vi "FindTag.vi"(8 "error in (no error)":errorcluster, 10 "Tag":string, 11 "ToolStripItem":refnum<k24>) -> (0 "error out":errorcluster, 2 "Found":bool, 3 "ToolStripItem out":refnum<k24>)   [LabVIEW 2016, in "MGI_MenuStrip.lvclass"]
doc: "Authored by Derek E. Trepanier\nsupport@mooregoodideas.com\nwww.mooregoodideas.com\n\nCopyright (c) 2012, Moore Good Ideas, Inc.\n\nAll rights reserved.\n\nRedistribution and use in source and binary forms, with or without modification, are permitted provided that the following conditions are met:\n\n * Redistributions of source code must retain the above copyright notice, this list of conditions and the following disclaimer.\n * Redistributions in binary form must reproduce the above copyright notice, this list of conditions and the following disclaimer in the documentation and/or other materials provided with the distribution.\n * Neither the name of Moore Good Ideas, Inc. nor the names of its contributors may be used to endorse or promote products derived from this software without specific prior written permission.\n\nTHIS SOFTWARE IS PROVIDED BY THE COPYRIGHT HOLDERS AND CONTRIBUTORS \"AS IS\" AND ANY EXPRESS OR IMPLIED WARRANTIES, INCLUDING, BUT NOT LIMITED TO, THE IMPLIED WARRANTIES OF MERCHANTABILITY AND FITNESS FOR A PARTICULAR PURPOSE ARE DISCLAIMED. IN NO EVENT SHALL THE COPYRIGHT OWNER OR CONTRIBUTORS BE LIABLE FOR ANY DIRECT, INDIRECT, INCIDENTAL, SPECIAL, EXEMPLARY, OR CONSEQUENTIAL DAMAGES (INCLUDING, BUT NOT LIMITED TO, PROCUREMENT OF SUBSTITUTE GOODS OR SERVICES; LOSS OF USE, DATA, OR PROFITS; OR BUSINESS INTERRUPTION) HOWEVER CAUSED AND ON ANY THEORY OF LIABILITY, WHETHER IN CONTRACT, STRICT LIABILITY, OR TORT (INCLUDING NEGLIGENCE OR OTHERWISE) ARISING IN ANY WAY OUT OF THE USE OF THIS SOFTWARE, EVEN IF ADVISED OF THE POSSIBILITY OF SUCH DAMAGE."
uses:
  <userlib>/_MGI/Menu Building/MenuTypes/MenuStrip/MGI_MenuStrip.lvclass
  System.Windows.Forms
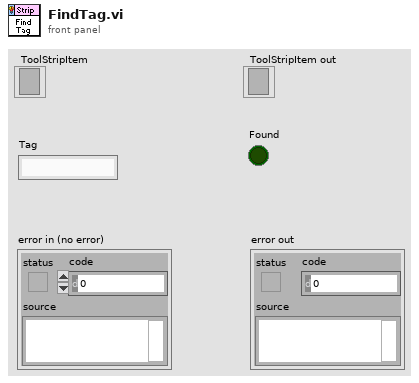
[diagram p1: front panel]
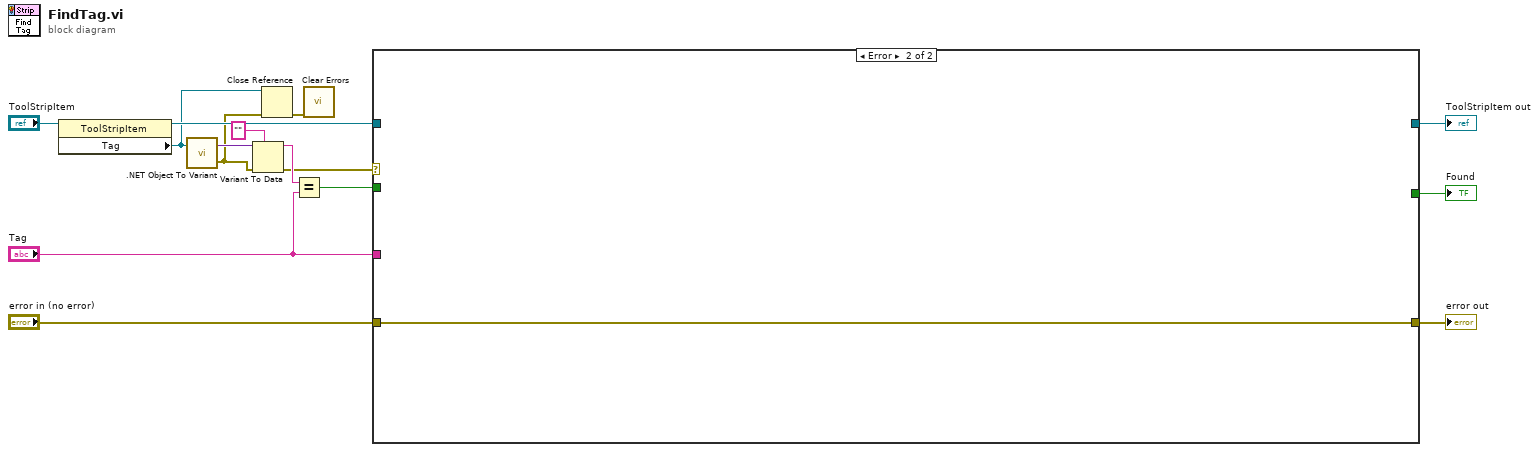
[diagram p0: block diagram]
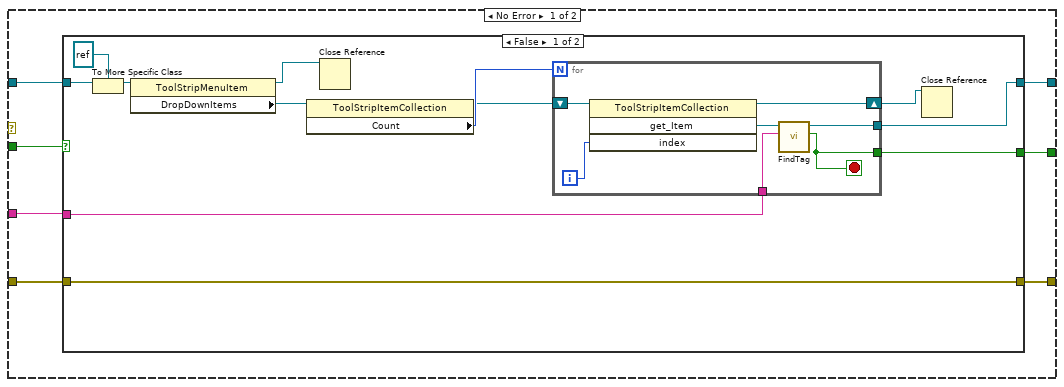
[diagram p2: hidden frame]
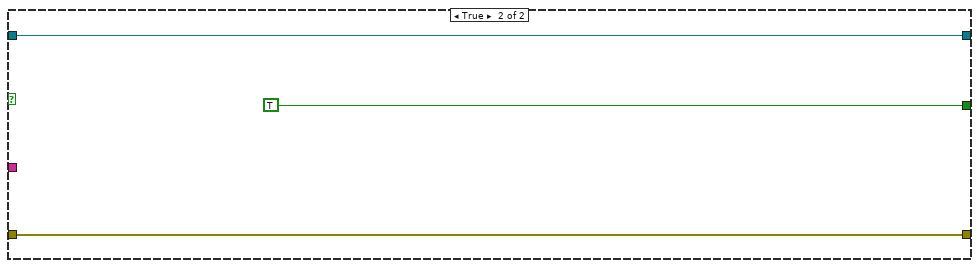
[diagram p3: hidden frame]
diagram:
  n1 = property class="ToolStripItem"(reference="ToolStripItem") -> (reference out=w9:refnum<k24>, "Tag"=w4:refnum<k24>)  [unwired: 1 in, 1 out]
  n2 = call <vilib>:".NET Object To Variant.vi"(".NET object"=w4) -> ("error out"=w3:errorcluster, "variant"=w14:variant)  [unwired: 1 in]
  n3 = Variant To Data(error in=w3, type="", Variant=w14) -> (data=w12:string, error out=w1:errorcluster)
  n4 = Close Reference(reference=w4, error in (no error)=w3) -> (error out=w2:errorcluster)
  n5 = Equal?(x=w12, y="Tag") -> (x = y?=w11:bool)
  n6 = call <vilib>:"Clear Errors.vi"("error in (no error)"=w2) -> ()  [unwired: 5 in, 2 out]
  n7 = case shown="Error" w1 {
    tunnel: w11 -> [w22 _]
    tunnel: [w21 _] -> w10
    tunnel: w9 -> [w20 _]
    tunnel: [w19 _] -> w8
    tunnel: [w18 w45] -> w7
    tunnel: "error in (no error)" -> [w17 w45]
    tunnel: "Tag" -> [w16 _]
    frame No Error {
      n8 = case shown="False" w22 {
        tunnel: [w27 w44] -> w21
        tunnel: w20 -> [w34 w44]
        tunnel: [w26 TRUE] -> w19
        tunnel: [w25 w42] -> w18
        tunnel: w17 -> [w25 w42]
        tunnel: w16 -> [w28 _]
        frame False {
          n9 = To More Specific Class(target class=refnum<k24> refnum ("new reference"), reference=w34) -> (specific class reference=w33:refnum<k24>)  [unwired: 1 in, 1 out]
          n10 = property class="ToolStripMenuItem"(reference=w33) -> (reference out=w23:refnum<k24>, "DropDownItems"=w31:refnum<k24>)  [unwired: 1 in, 1 out]
          n11 = property class="ToolStripItemCollection"(reference=w31) -> (reference out=w29:refnum<k24>, "Count"=w30:i32)  [unwired: 1 in, 1 out]
          n12 = Close Reference(reference=w23) -> ()  [unwired: 1 in, 1 out]
          n13 = for {
            N: w30 -> [_]
            tunnel: w28 -> [w38]
            tunnel: [w37] -> w27
            tunnel: [w36] -> w26
            shift-right: [w35] -> w24
            shift-left: w29 -> [w41]
            i -> [w40]
            stop <- w36 stop-if-true
            n14 = invoke class="ToolStripItemCollection" method="get_Item"(reference=w41, "index"=w40) -> (reference out=w35:refnum<k24>, "get_Item"=w39:refnum<k24>)  [unwired: 2 in, 2 out]
            n15 = call <userlib>:"FindTag.vi"("Tag"=w38, "ToolStripItem"=w39) -> ("Found"=w36:bool, "ToolStripItem out"=w37:refnum<k24>)  [unwired: 7 in, 1 out]
          }
          n16 = Close Reference(reference=w24) -> ()  [unwired: 1 in, 1 out]
        }
        frame True {
        }
      }
    }
    frame Error {
    }
  }
  "error out" <- w7
  "ToolStripItem out" <- w10
  "Found" <- w8
